vi "I2C.WriteByteArray.vi"(5 "I2C Address":u16 format="%x", 7 "I2C Register":u16 format="%x", 8 "error in":errorcluster, 9 "DownloadChunkSize":u8=30, 10 "I2C Write Data":u8[](array[numeric]), 11 "comport in":refnum<visa-resource-name>) -> (0 "error out":errorcluster, 1 "WrittenBytes":i32, 3 "comport out":refnum<visa-resource-name>)   [LabVIEW 2020, in "FirmataClient.lvlib"]
doc: "Transmit a byte array to the UUT for a target I2C device running on its board"
uses:
  FirmataClient.lvlib
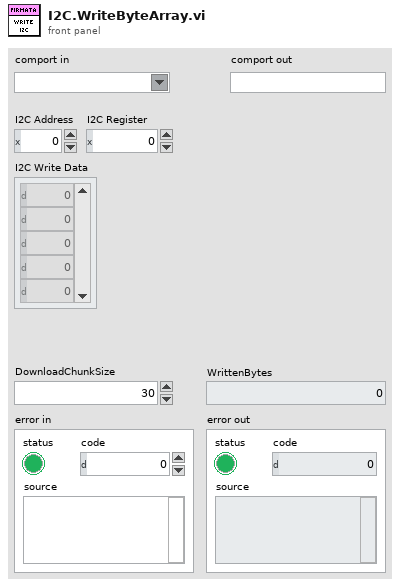
[diagram p1: front panel]
types:
  T1 = enum16{"Write", "Read Once", "Read Continuously", "Stop Continuous Reading"}
  T2 = typedef "FirmataClient.lvlib/FirmataProtocolConstants.ctl" = u16
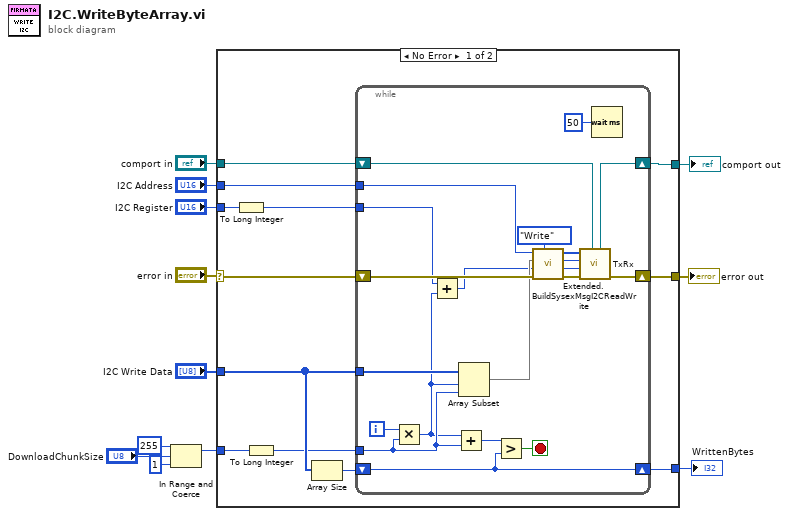
[diagram p0: block diagram]
diagram:
  n1 = In Range and Coerce(upper limit=u8 255, x="DownloadChunkSize", lower limit=u8 1) -> (coerced(x)=w5:u8)  [unwired: 1 out]
  n2 = case shown="No Error" "error in" {
    selector: "error in" -> [w22 w47]
    tunnel: [w20 w47] -> w11
    tunnel: [w24 w46] -> w7
    tunnel: "comport in" -> [w23 w46]
    tunnel: "I2C Address" -> [w21 _]
    tunnel: "I2C Register" -> [w14 _]
    tunnel: w5 -> [w16 _]
    tunnel: [w18 _] -> w2
    tunnel: "I2C Write Data" -> [w17 _]
    frame No Error {
      n3 = To Long Integer(number=w14) -> (32bit integer=w13:i32)
      n4 = To Long Integer(number=w16) -> (32bit integer=w15:i32)
      n5 = Array Size(array=w17) -> (size(s)=w19:i32)
      n6 = while {
        tunnel: w21 -> [w30]
        tunnel: w17 -> [w36]
        tunnel: w13 -> [w29]
        shift-right: [w41] -> w24
        shift-left: w23 -> [w40]
        shift-right: [w38] -> w20
        shift-left: w22 -> [w39]
        tunnel: w15 -> [w33]
        shift-right: [w26] -> w18
        shift-left: w19 -> [w26]
        i -> [w34]
        stop <- w31 stop-if-true
        n7 = Multiply(x=w34, y=w33) -> (x*y=w28:i32)
        n8 = Add(x=w29, y=w28) -> (x+y=w27:i32)
        n9 = Add(x=w28, y=w33) -> (x+y=w32:i32)
        n10 = Array Subset(array=w36, index=w28, length=w33) -> (w35:u8[])
        n11 = Greater?(x=w32, y=w26) -> (0:w31:bool)
        n12 = call "Extended.BuildSysexMsgI2CReadWrite.vi"("Read/Write Mode"=T1."Write", "error in"=w39, "Register"=w27, "I2C Write Data"=w35, "Slave Address"=w30) -> ("error out"=w45:errorcluster, "ReplyLength"=w42:i32, "ReplyFirstByte"=w43:T2, "I2CRequestMessage"=w44:u8[])  [unwired: 3 in]
        n13 = call "TxRx.vi"("comport in"=w40, "error in"=w45, "Expected Reply Length"=w42, "ReplyFirstByte"=w43, "MessageToSend"=w44) -> ("error out"=w38:errorcluster, "comport out"=w41:refnum<visa-resource-name>)  [unwired: 2 in, 3 out]
        n14 = Wait (ms)(milliseconds to wait=u32 50) -> ()  [unwired: 1 out]
      }
    }
    frame Error {
    }
  }
  "error out" <- w11
  "comport out" <- w7
  "WrittenBytes" <- w2
